vi "Colour -电机.vi"(9 "result":string, 11 "colourRef":refnum<vi>) -> (3 "colourRef 2":refnum<vi>)   [LabVIEW 2020]
uses:
  Global_Variable/Global.vi
panel:
  out "错误输出":errorcluster
  in  "字符串":string="黄"
  in  "result 2":string
  in  "黄灯":bool
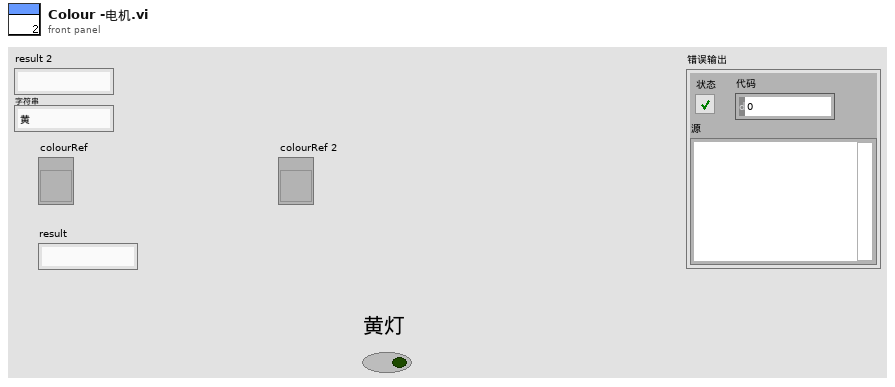
[diagram p1: front panel]
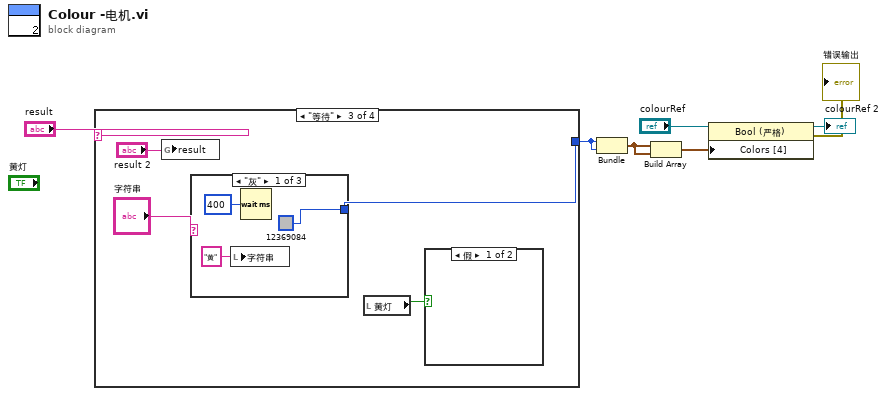
[diagram p0: block diagram]
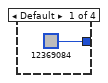
[diagram p2: hidden frame]
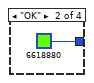
[diagram p3: hidden frame]
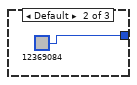
[diagram p4: hidden frame]
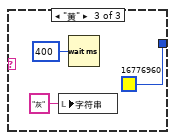
[diagram p5: hidden frame]
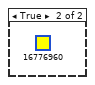
[diagram p6: hidden frame]
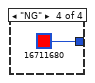
[diagram p7: hidden frame]
diagram:
  n1 = case shown="\"等待\"" "result" {
    tunnel: [u32 12369084 u32 6618880 w10 u32 16711680] -> w7
    frame Default {
    }
    frame "OK" {
    }
    frame "等待" {
      n2 = global write "Global.vi" "result"("result 2") -> ()
      n3 = case shown="\"灰\"" "字符串" {
        tunnel: [u32 12369084 u32 12369084 u32 16776960] -> w10
        frame "灰" {
          n4 = local write "字符串"("黄" ("字符串")) -> ()
          n5 = Wait (ms)(milliseconds to wait=u32 400 ("等待时间（毫秒）")) -> ()  [unwired: 1 out]
        }
        frame Default {
        }
        frame "黄" {
          n6 = local write "字符串"("灰" ("字符串")) -> ()
          n7 = Wait (ms)(milliseconds to wait=u32 400 ("等待时间（毫秒）")) -> ()  [unwired: 1 out]
        }
      }
      n8 = local read "黄灯"() -> (w13:bool)
      n9 = case shown="假" w13 {
        frame False {
        }
        frame True {
          (unwired) u32 16776960
        }
      }
    }
    frame "NG" {
    }
  }
  n10 = Bundle(w7, w7) -> (w6:cluster{u32, u32})  [unwired: 1 in]
  n11 = Build Array(w6, w6) -> (w2:cluster{u32, u32}[])
  n12 = property class="Bool (严格)"(reference="colourRef", "Colors [4]"=w2) -> (reference out=→"colourRef 2":refnum<vi>, error out=→"错误输出":errorcluster)  [unwired: 1 in]
